vi "Get Picture Ring Images From Variables.vi"(8 "error in (no error)":errorcluster, 10 "Ring Image Variable Name":string, 11 "Web FP In":refnum<class "Web Front Panel.lvclass">) -> (0 "error out":errorcluster, 3 "Images":string[](array[string]))   [LabVIEW 2015, in "Front Panel Publisher.lvlib" / "Web Front Panel.lvclass"]
uses:
  Web Front Panel.lvclass
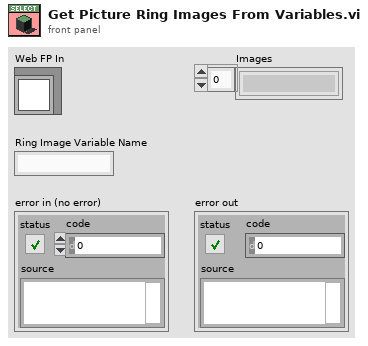
[diagram p1: front panel]
types:
  T1 = typedef "Front Panel Publisher.lvlib/Web Front Panel.lvclass/Object Attributes.ctl" = cluster{"VI Name":string, "VI Reference":refnum<vi>, "Controls":refnum<class "Object.lvclass">[], "Indicators":refnum<class "Object.lvclass">[], "Decorations":refnum<class "Object.lvclass">[], "VR With Previous Get":refnum<data-value>, "VR With Ring Images":refnum<data-value>}
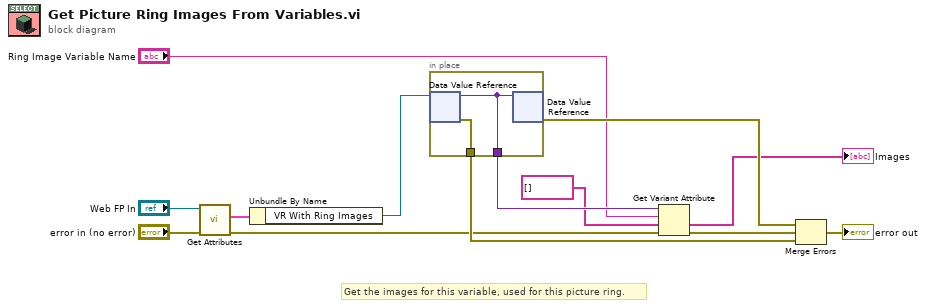
[diagram p0: block diagram]
diagram:
  # "Get the images for this variable, used for this picture ring."
  n1 = call "Get Attributes.vi"("error in (no error)"="error in (no error)", "Web FP In"="Web FP In") -> ("error out"=w2:errorcluster, "Data"=w10:T1)  [unwired: 6 in, 2 out]
  n2 = Unbundle By Name(w10) -> ("VR With Ring Images"=w12:refnum<data-value>)
  n3 = in-place {
    in-place-border: [w15] -> w6
    in-place-border: [w14] -> w8
    n4 = in-place-dvr #1(w12) -> (w15:variant, w14:errorcluster)
    n5 = in-place-dvr #1(w15) -> (w7:errorcluster)  [unwired: 1 out]
  }
  n6 = Get Variant Attribute(Variant=w6, name="Ring Image Variable Name", default value (empty Variant)=string[] [], error in=w2) -> (value=→"Images":string[], error out=w1:errorcluster)  [unwired: 2 out]
  n7 = Merge Errors(w7, w1, w8) -> (→"error out":errorcluster)
